vi "read_BLUEFORS_Temperatures_JSON.vi"(7 "Web(T)":bool=TRUE, 8 "Error In":errorcluster, 11 "url":string="http://192.168.0.101:5001/channel/measurement/latest") -> (0 "Error Out":errorcluster, 1 "temperatura":dbl, 2 "chan_nr":i32, 3 "date/time string":string, 4 "STATUS":string, 5 "datoNuevo?":bool=TRUE)   [LabVIEW 2017]
uses:
  datos_BLUEFORS.ctl
  <vilib>/httpClient/LabVIEWHTTPClient.lvlib
panel:
  out "value":T1
  out "Datos":string[](array[string])
  out "Cabecera":string[](array[string])
  out "datos BLUEFORS":T2 {"imz" format="%.3f"; "status_flags" format="%.3f"; "magnitude" format="%.3f"; "reactance" format="%.3f"; "datetime" format="%.3f"; "channel_nr" format="%.3f"; "resistance" format="%.3f"; "timestamp" format="%.3f"; "settings_nr" format="%.3f"; "temperature" format="%.3f"; "angle" format="%.3f"; "status" format="%.3f"; "rez" format="%.3f"}
  out "body":string="{\"rez\": 178.573, \"status\": \"OK\", \"angle\": 90.054, \"temperature\": 4.268984, \"settings_nr\": 17, \"timestamp\": 1655726623.39446, \"resistance\": 178.573, \"channel_nr\": 5, \"datetime\": \"2022-06-20T12:03:55.010794Z\", \"reactance\": -186159.948, \"magnitude\": 178.573, \"status_flags\": [], \"imz\": -0.171}"
  out "headers":string="HTTP/1.1 200 OK\r\nContent-Length: 271\r\nServer: TornadoServer/5.1.1\r\nEtag: \"846106313589bc8d9fa2b11791fa3e2bef692078\"\r\nDate: Wed, 09 Jun 2021 16:16:40 GMT\r\nAccess-Control-Allow-Origin: *\r\nAccess-Control-Allow-Headers: access-control-allow-origin,authorization,content-type\r\nContent-Type: application/json; charset=UTF-8\r\n\r\n"
  # "LEE EL FICHERO TXT ALMACENADO EN EL SERVIDOR WEB\nEXTRAE LOS VALORES ORDENADOS A UNA MATRIZ"
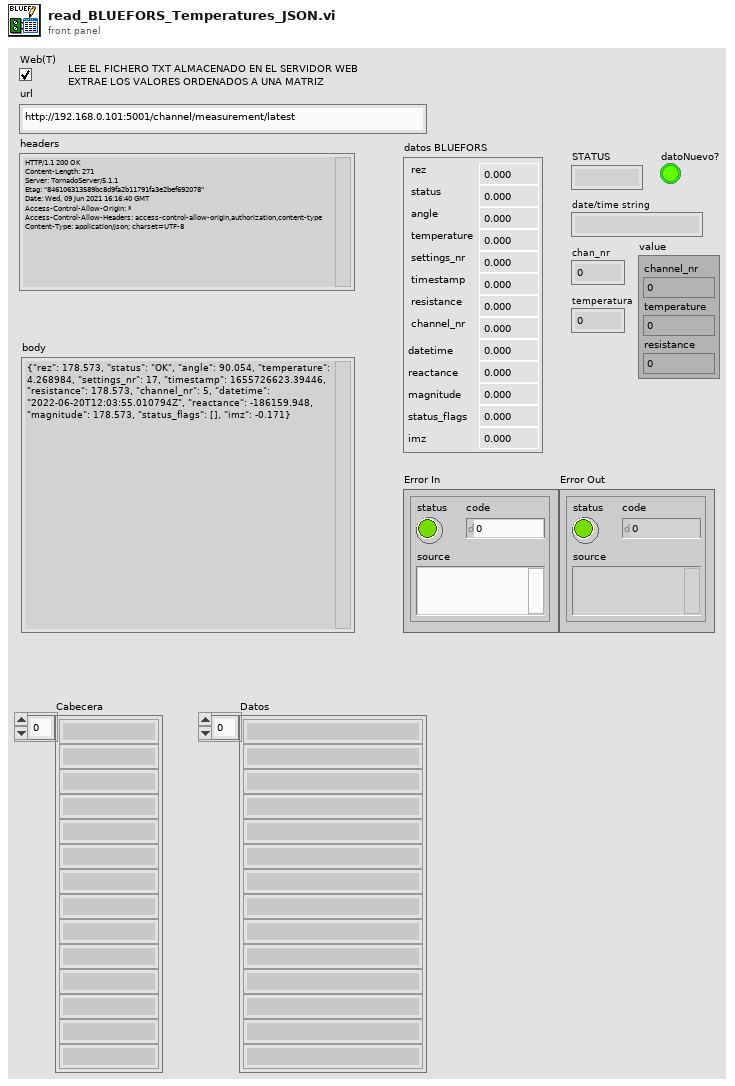
[diagram p1: front panel]
types:
  T1 = cluster{"channel_nr":i32, "temperature":dbl, "resistance":dbl}
  T2 = typedef "datos_BLUEFORS.ctl" = cluster{"rez":dbl, "status":dbl, "angle":dbl, "temperature":dbl, "settings_nr":dbl, "timestamp":dbl, "resistance":dbl, "channel_nr":dbl, "datetime":dbl, "reactance":dbl, "magnitude":dbl, "status_flags":dbl, "imz":dbl}
  T3 = typedef "LabVIEWHTTPClient.lvlib/ClientHandle.ctl" = refnum<k1>
  T4 = cluster{"heater_nr":i32, "target_temperature":dbl, "power":dbl}
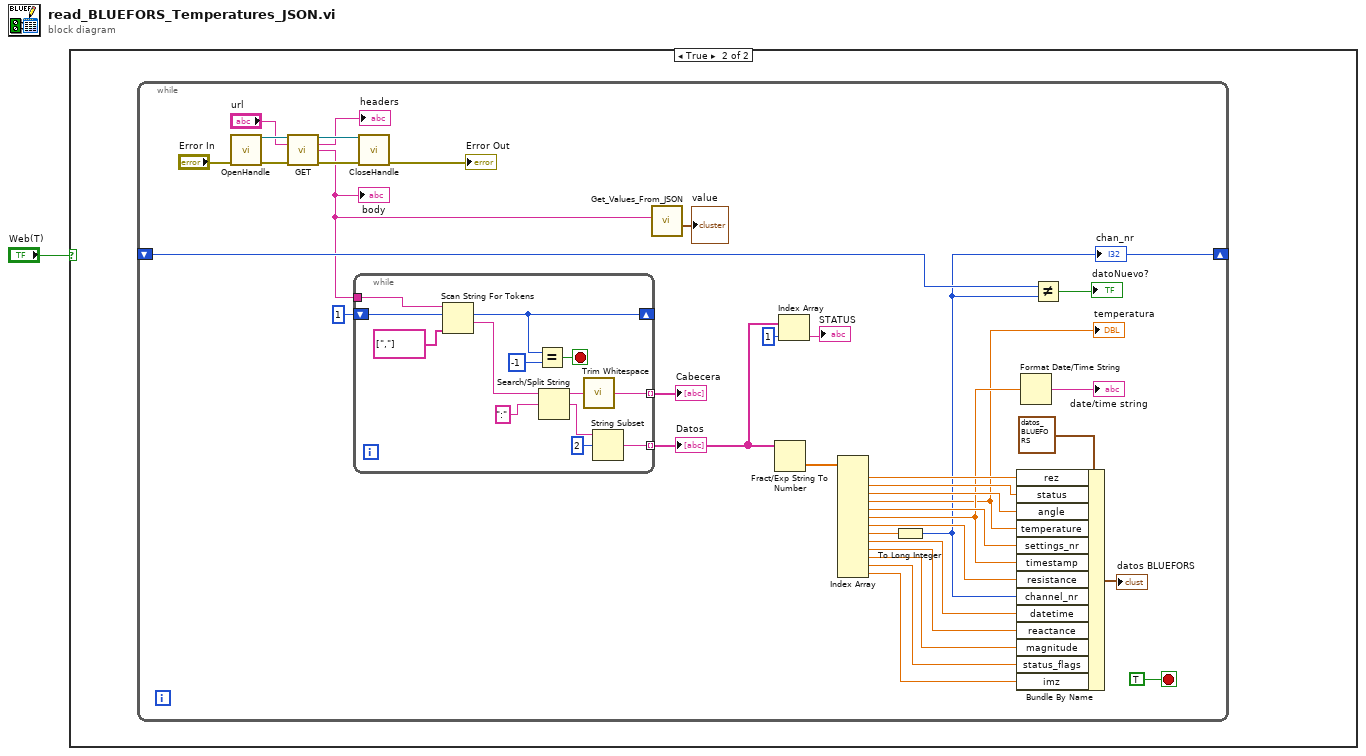
[diagram p0: block diagram]
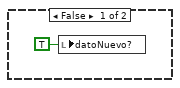
[diagram p2: hidden frame]
diagram:
  n1 = case shown="True" "Web(T)" {
    frame False {
      n2 = local write "datoNuevo?"(TRUE ("datoNuevo?")) -> ()
    }
    frame True {
      n3 = while {
        shift-right: [w6] -> _
        shift-left: _ -> [w32]
        stop <- TRUE stop-if-true
        n4 = call <vilib>:"OpenHandle.vi"("error in (no error)"="Error In") -> ("client handle out"=w29:T3, "error out"=w25:errorcluster)  [unwired: 13 in]
        n5 = call <vilib>:"GET.vi"("client handle"=w29, "url"="url", "error in (no error)"=w25) -> ("client handle out"=w28:T3, "headers"=→"headers":string, "body"=w3:string, "error out"=w26:errorcluster)  [unwired: 9 in]
        "body" <- w3
        n6 = while {
          tunnel: w3 -> [w51]
          shift-right: [w46] -> _
          shift-left: 1 ("offset past token") -> [w49]
          tunnel: [w42] -> w34 mode=indexing
          tunnel: [w40] -> w4 mode=indexing
          stop <- w48 stop-if-true
          n7 = Scan String For Tokens(6:string[] [","] ("operators (none)"), 8:w49, 9:w51) -> (1:w45:string, 2:w46:i32)  [unwired: 3 in, 2 out]
          n8 = Equal?(x=w46, y=-1) -> (x = y?=w48:bool)
          n9 = Search/Split String(string=w45, search string/char (-)=":" ("element")) -> (substring before match=w43:string, match + rest of string=w41:string)  [unwired: 1 in, 1 out]
          n10 = call <vilib>:"Trim Whitespace.vi"("string"=w43) -> ("trimmed string"=w42:string)  [unwired: 1 in]
          n11 = String Subset(string=w41, offset (0)=2) -> (substring=w40:string)  [unwired: 1 in]
        }
        "Cabecera" <- w34
        "Datos" <- w4
        n12 = call <vilib>:"CloseHandle.vi"("client handle"=w28, "error in (no error)"=w26) -> ("error out"=→"Error Out":errorcluster)  [unwired: 13 in]
        n13 = call "Get_Values_From_JSON.vi"("utf-8 text"=w3) -> ("value"=→"value":T4)  [unwired: 9 in, 1 out]
        n14 = Fract/Exp String To Number(string=w4) -> (number=w33:dbl[])  [unwired: 3 in, 1 out]
        n15 = Index Array(array=w4, index=1) -> (element=→"STATUS":string)
        n16 = Index Array(array=w33) -> (element #1=w22:dbl, element #2=w19:dbl, element #3=w18:dbl, element #4=w7:dbl, element #5=w17:dbl, element #6=w10:dbl, element #7=w16:dbl, element #8=w8:dbl, element #9=w15:dbl, element #10=w14:dbl, element #11=w13:dbl, element #12=w12:dbl, element #13=w11:dbl)  [unwired: 13 in]
        "temperatura" <- w7
        n17 = To Long Integer(number=w8) -> (32bit integer=w6:i32)
        "chan_nr" <- w6
        n18 = Bundle By Name(cluster=T2 {"rez"=93.296, "status"=0.0, "angle"=90.069, "temperature"=25.905019, "settings_nr"=0.0, "timestamp"=0.0, "resistance"=1655898328.20644, "channel_nr"=93.296, "datetime"=0.0, "reactance"=0.0, "magnitude"=-76836.555, "status_flags"=0.0, "imz"=0.0} ("datos BLUEFORS"), "rez"=w22, "status"=w19, "angle"=w18, "temperature"=w7, "settings_nr"=w17, "timestamp"=w10, "resistance"=w16, "channel_nr"=w6, "datetime"=w15, "reactance"=w14, "magnitude"=w13, "status_flags"=w12, "imz"=w11) -> (→"datos BLUEFORS":T2)
        n19 = Format Date/Time String(seconds (now)=w10) -> (date/time string=→"date/time string":string)  [unwired: 2 in]
        n20 = Not Equal?(x=w32, y=w6) -> (x != y?=→"datoNuevo?":bool)
      }
    }
  }
